vi "disable_Config.vi"() -> ()   [LabVIEW 2014]
uses:
  aardvark.dll
panel:
  in  "Aardvark Handle":i32 min=0
  out "Data Written":bool
  in  "Num Bytes to Fetch (64)":u8=64 min=1
  out "error out":errorcluster
  in  "Address (0x50)":u16=80 max=1023 format="%.0x"
  in  "error in (no error)":errorcluster
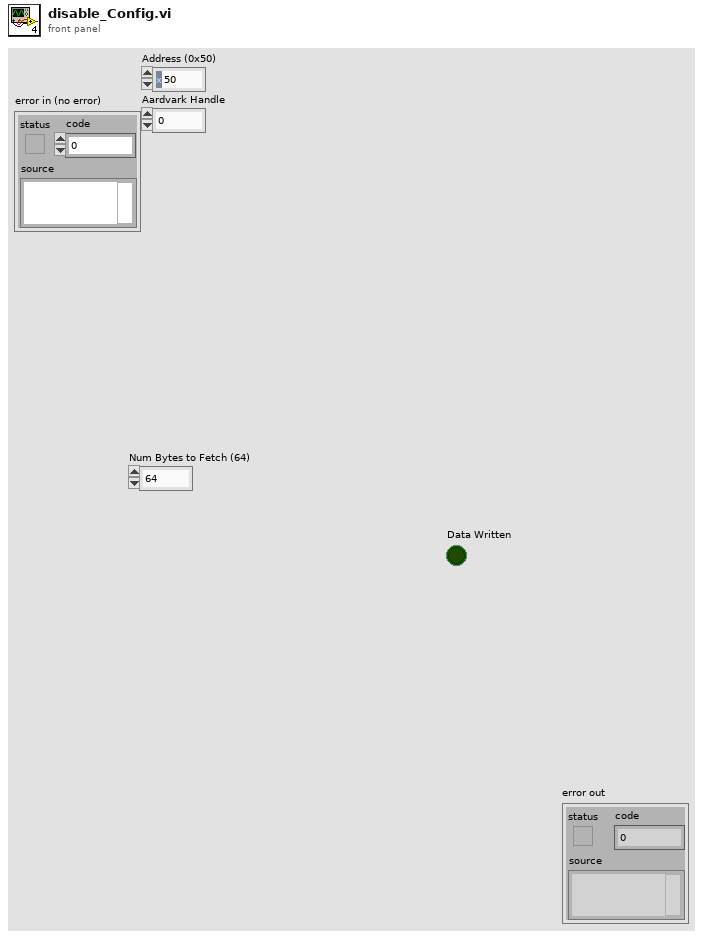
[diagram p1: front panel]
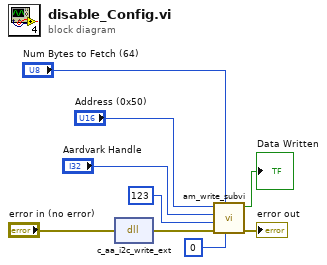
[diagram p0: block diagram]
diagram:
  n1 = dll-call lib="C:/Users/p282652/Documents/LabVIEW Data/Demonstrator/labviewFunctions_AM/aardvark.dll" fn="c_aa_i2c_write_ext"(error in="error in (no error)") -> (error out=w7:errorcluster)  [unwired: 3 in, 1 out]
  n2 = call "am_write_subvi.vi"("Data to Write"=u8 0, "Num Bytes to Fetch (64)"="Num Bytes to Fetch (64)", "error in (no error)"=w7, "Memory ADD"=u8 123, "Aardvark Handle in"="Aardvark Handle", "Address (0x50) in"="Address (0x50)") -> ("error out"=→"error out":errorcluster, "Data Written"=→"Data Written":bool)  [unwired: 4 in]
